vi "4 Way Sub.vi"(3 "OldVal":T1) -> (1 "Mode Select":enum8{"Off", "Stby", "Hold", "Run"}(ring))   [LabVIEW 2012]
uses:
  Type Defs/4 Way Button.ctl
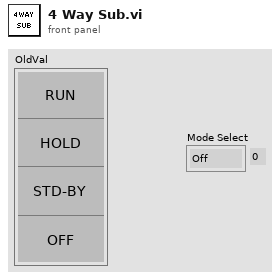
[diagram p1: front panel]
types:
  T1 = typedef "4 Way Button.ctl" = cluster{"Off":bool, "Standby":bool, "Hold":bool, "Run":bool}
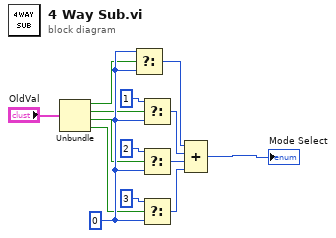
[diagram p0: block diagram]
diagram:
  w11 = u8 0 ("f")
  n1 = Unbundle("OldVal") -> ("Off"=w3:bool, "Standby"=w4:bool, "Hold"=w5:bool, "Run"=w6:bool)
  n2 = Select(t=w11, s=w3, f=w11) -> (s? t:f=w7:u8)
  n3 = Select(t=u8 1, s=w4, f=w11) -> (s? t:f=w8:u8)
  n4 = Select(t=u8 2, s=w5, f=w11) -> (s? t:f=w9:u8)
  n5 = Select(t=u8 3, s=w6, f=w11) -> (s? t:f=w10:u8)
  n6 = Compound Arithmetic op=ADD(w7, w8, w9, w10) -> (→"Mode Select":u8)
